vi "ZF Excel Read.vi"() -> ()   [LabVIEW 2021]
uses:
  <vilib>/Utility/file.llb/Read Delimited Spreadsheet (string).vi
panel:
  in  "Read Data":bool
  out "Read Data":cluster{"Value 1":dbl, "Message":string}[](array[cluster])
  in  "Array":cluster{"Value 1":dbl, "Message":string}[](array[cluster])
  # "Data Read to LabView from Excel"
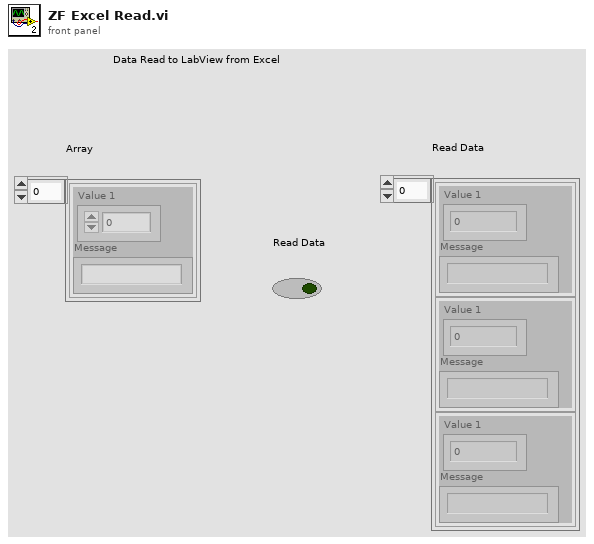
[diagram p1: front panel]
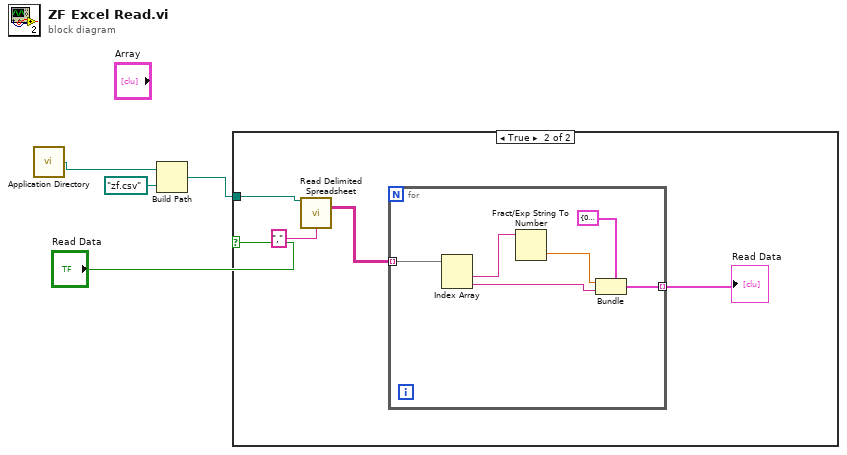
[diagram p0: block diagram]
diagram:
  n1 = call <vilib>:"Application Directory.vi"() -> ("Application Directory"=w4:path)
  n2 = Build Path(base path=w4, name or relative path=path "zf.csv") -> (appended path=w1:path)
  n3 = case shown="True" "Read Data" {
    tunnel: w1 -> [_ w8]
    frame False {
    }
    frame True {
      n4 = call-poly <vilib>:"Read Delimited Spreadsheet.vi"("file path (dialog if empty)"=w8, "delimiter (\\t)"="," ("delimiter (\\t)")) -> ("all rows"=w6:string[][])  [unwired: 8 in, 5 out]
      n5 = for {
        tunnel: w6 -> [w14] mode=indexing
        tunnel: [w12] -> w5 mode=indexing
        n6 = Index Array(array=w14) -> (element #1=w13:string, element #2=w10:string)  [unwired: 2 in]
        n7 = Fract/Exp String To Number(string=w13) -> (number=w11:dbl)  [unwired: 3 in, 1 out]
        n8 = Bundle(cluster=cluster{dbl, "String":string} {0.0, "String"=""}, w11, "String"=w10) -> (w12:cluster{dbl, "String":string})
      }
      "Read Data" <- w5
    }
  }
